vi "FTW-BuildUtil-PreBuild Action-Clean.vi"(6 "Top Level/Always Included VIs":path[](array[path]), 7 "Main Destination Path":path, 9 "Target Name":string, 10 "Build Specification Name":string, 11 "Project Path":path) -> (0 "error out":errorcluster)   [LabVIEW 2018]
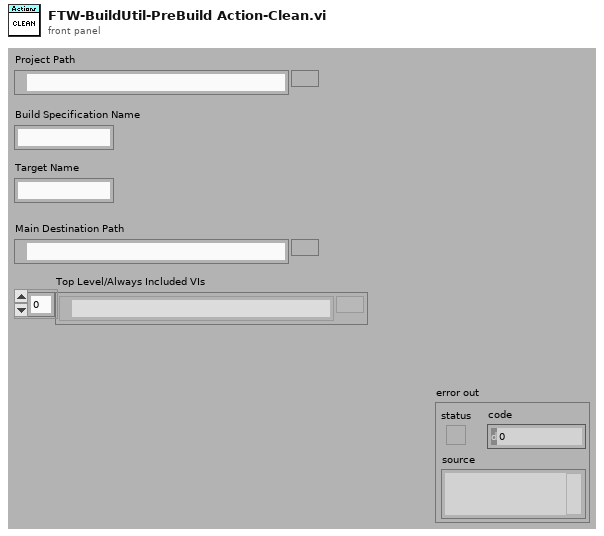
[diagram p1: front panel]
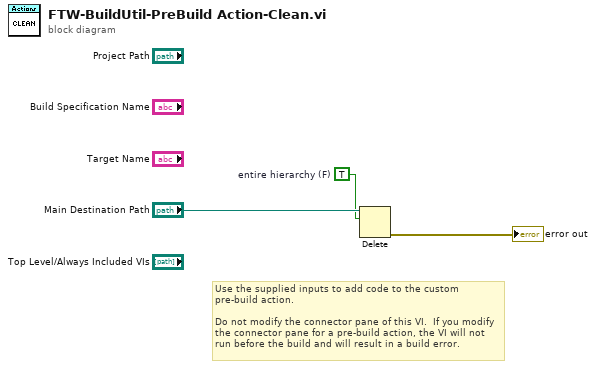
[diagram p0: block diagram]
diagram:
  w2 = TRUE  # entire hierarchy (F)
  # "Use the supplied inputs to add code to the custom pre-build action.\n\nDo not modify the connector pane of this VI.  If you modify the connector pane for a pre-build action, the VI will not run before the build and will result in a build error."
  n1 = Delete(path (use dialog)="Main Destination Path", entire hierarchy (F)=w2) -> (error out=→"error out":errorcluster)  [unwired: 3 in, 2 out]
